vi "Test.vi"() -> ()   [LabVIEW 2022 SP3, in "TcpServer.lvlib"]
uses:
  TcpServer.lvlib
  <vilib>/ActorFramework/Actor/Actor.lvclass
  TcpServer/TcpServer.lvclass
  <vilib>/ActorFramework/Stop Msg/Stop Msg.lvclass
  <vilib>/ActorFramework/Report Error Msg/Report Error Msg.lvclass
  TcpServer Messages/ServerStart Msg/ServerStart Msg.lvclass
  TcpServer Messages/ServerStop Msg/ServerStop Msg.lvclass
  TcpServer Messages/ServerConfig Msg/ServerConfig Msg.lvclass
  ServerConfig/ServerConfig.lvclass
  C:/Users/jakub/repos/gh/sw4sys/lv-tcp-server-sample/LoggingActor/Source/LoggingActor/LoggingActor/LoggingActor.lvclass
  C:/Program Files (x86)/National Instruments/LabVIEW 2022/vi.lib/ActorFramework/Actor/Actor.lvclass
  C:/Users/jakub/repos/gh/sw4sys/lv-tcp-server-sample/TcpServerSample/Source/TcpServerSample/TcpServer/TcpServer/TcpServer.lvclass
  C:/Users/jakub/repos/gh/sw4sys/lv-tcp-server-sample/TcpServerSample/Source/TcpServerSample/Connection/CallerMessage/CallerMessage.lvclass
panel:
  in  "Server Config":T1={"Address"="127.0.0.1", "Port"=0, "ReadMode"=enum."Standard", "OpenTimeout"=5000, "ReadTimeout"=5000, "WriteTimeout"=5000, "ConnectionTimeout"=5000}
  in  "BtnServerStop":bool
  in  "BtnServerStart":bool
  out "error out":errorcluster
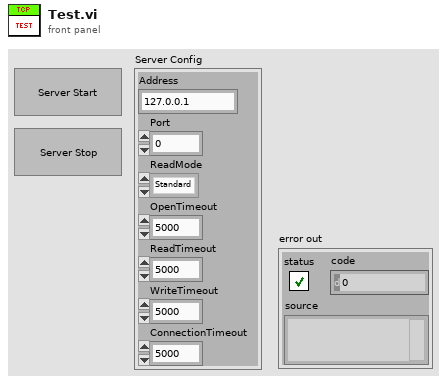
[diagram p1: front panel]
types:
  T1 = cluster{"Address":string, "Port":u16, "ReadMode":enum16{"Standard", "Buffered", "CRLF", "Immediate"}, "OpenTimeout":i32, "ReadTimeout":i32, "WriteTimeout":i32, "ConnectionTimeout":i32}
  T2 = enum16{"Standard", "Buffered", "CRLF", "Immediate"}
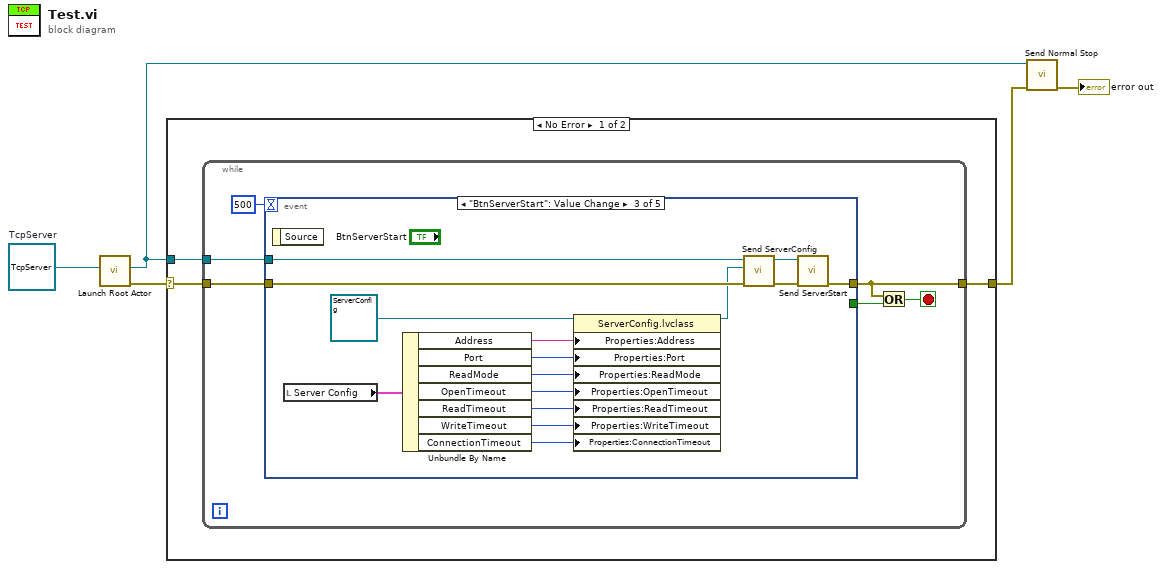
[diagram p0: block diagram]
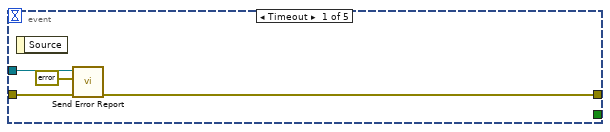
[diagram p2: hidden frame]
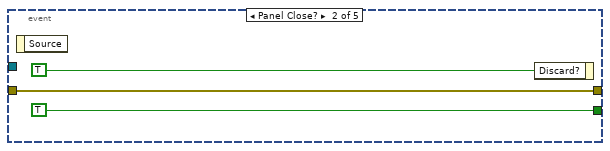
[diagram p3: hidden frame]
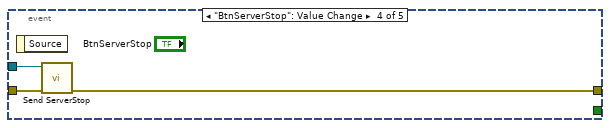
[diagram p4: hidden frame]
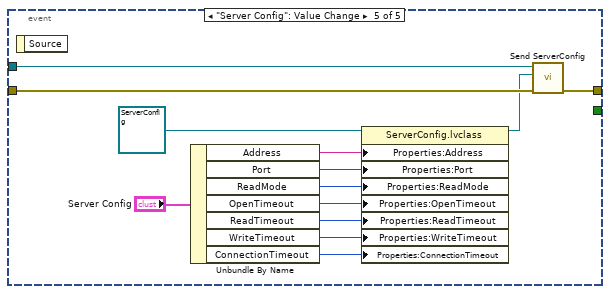
[diagram p5: hidden frame]
diagram:
  w5 = refnum<class "TcpServer.lvclass"> refnum  # TcpServer
  n1 = call <vilib>:"Launch Root Actor.vi"("Actor"=w5) -> ("error out"=w4:errorcluster, "Actor's Enqueuer"=w1:refnum<class "Message Enqueuer.lvclass">)  [unwired: 9 in]
  n2 = case shown="No Error" w4 {
    selector: w4 -> [w8 w53]
    tunnel: w1 -> [w7 _]
    tunnel: [w6 w53] -> w3
    frame No Error {
      n3 = while {
        tunnel: w7 -> [w13]
        tunnel: w8 -> [w14]
        tunnel: [w9] -> w6
        stop <- w11 stop-if-true
        n4 = event shown="[2] \"BtnServerStart\": Value Change" {
          selector: _ -> [_ _ _ _ _]
          dyn-events: _ -> [_ _ _ _ _]
          timeout: 500 -> [_ _ _ _ _]
          tunnel: [_ TRUE ("Discard?") _ _ _] -> w10
          tunnel: w14 -> [w17 w20 w36 w38 w52]
          tunnel: [w18 w20 w35 w37 w50] -> w9
          tunnel: w13 -> [w16 _ w33 w39 w51]
          event Timeout {
            n5 = event-data() -> ()  [unwired: 1 in, 1 out]
            n6 = call <vilib>:"Send Error Report.vi"("error in (no error)"=w17, "Error From Sender"=errorcluster {"status"=FALSE, "code"=0, "source"=""}, "Message Enqueuer"=w16) -> ("error out"=w18:errorcluster)  [unwired: 8 in]
          }
          event Panel Close? {
            n7 = event-data() -> ()  [unwired: 1 in, 1 out]
            n8 = event-data("Discard?"=TRUE) -> ()  [unwired: 1 in, 1 out]
          }
          event "BtnServerStart": Value Change {
            n9 = event-data() -> ()  [unwired: 1 in, 1 out]
            n10 = local read "Server Config"() -> (w24:T1)
            n11 = Unbundle By Name(w24) -> ("Address"=w30:string, "Port"=w29:u16, "ReadMode"=w28:T2, "OpenTimeout"=w27:i32, "ReadTimeout"=w26:i32, "WriteTimeout"=w25:i32, "ConnectionTimeout"=w22:i32)
            n12 = property class="ServerConfig.lvclass"(reference=refnum<class "ServerConfig.lvclass"> refnum ("ServerConfig"), "Properties:Address"=w30, "Properties:Port"=w29, "Properties:ReadMode"=w28, "Properties:OpenTimeout"=w27, "Properties:ReadTimeout"=w26, "Properties:WriteTimeout"=w25, "Properties:ConnectionTimeout"=w22) -> (reference out=w23:refnum<class "ServerConfig.lvclass">)  [unwired: 1 in, 1 out]
            n13 = call "Send ServerConfig.vi"("error in (no error)"=w36, "ServerConfig"=w23, "Message Enqueuer"=w33) -> ("error out"=w34:errorcluster, "Message Enqueuer out"=w32:refnum<class "Message Enqueuer.lvclass">)  [unwired: 7 in]
            n14 = call "Send ServerStart.vi"("error in (no error)"=w34, "Message Enqueuer"=w32) -> ("error out"=w35:errorcluster)  [unwired: 8 in, 1 out]
          }
          event "BtnServerStop": Value Change {
            n15 = event-data() -> ()  [unwired: 1 in, 1 out]
            n16 = call "Send ServerStop.vi"("error in (no error)"=w38, "Message Enqueuer"=w39) -> ("error out"=w37:errorcluster)  [unwired: 8 in, 1 out]
          }
          event "Server Config": Value Change {
            n17 = event-data() -> ()  [unwired: 1 in, 1 out]
            n18 = Unbundle By Name("Server Config") -> ("Address"=w46:string, "Port"=w45:u16, "ReadMode"=w44:T2, "OpenTimeout"=w43:i32, "ReadTimeout"=w42:i32, "WriteTimeout"=w41:i32, "ConnectionTimeout"=w40:i32)
            n19 = property class="ServerConfig.lvclass"(reference=refnum<class "ServerConfig.lvclass"> refnum ("ServerConfig"), "Properties:Address"=w46, "Properties:Port"=w45, "Properties:ReadMode"=w44, "Properties:OpenTimeout"=w43, "Properties:ReadTimeout"=w42, "Properties:WriteTimeout"=w41, "Properties:ConnectionTimeout"=w40) -> (reference out=w48:refnum<class "ServerConfig.lvclass">)  [unwired: 1 in, 1 out]
            n20 = call "Send ServerConfig.vi"("error in (no error)"=w52, "ServerConfig"=w48, "Message Enqueuer"=w51) -> ("error out"=w50:errorcluster)  [unwired: 7 in, 1 out]
          }
        }
        n21 = Or(x=w9, y=w10) -> (x .or. y?=w11:bool)
      }
    }
    frame Error {
    }
  }
  n22 = call <vilib>:"Send Normal Stop.vi"("error in (no error)"=w3, "Message Enqueuer"=w1) -> ("error out"=→"error out":errorcluster)  [unwired: 9 in]
